vi "Burning Queue.vi"() -> (0 "error out 2":errorcluster)   [LabVIEW 2022 SP3]
uses:
  Type Def/Burning States.ctl
panel:
  in  "error in (no error)":errorcluster
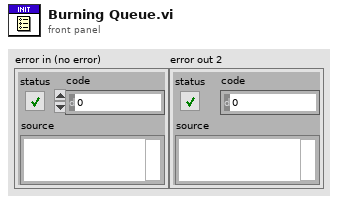
[diagram p1: front panel]
types:
  T1 = typedef "Burning States.ctl" = enum16{"Open Ports", "Close Ports", "Main", "Settings", "Voltaje", "Probe", "Lenguaje", "Callibration", "Exit", "Voltage Test", "Test 2", "End test"}
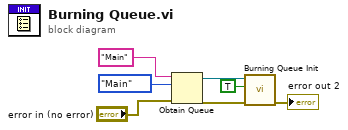
[diagram p0: block diagram]
diagram:
  n1 = Obtain Queue(name (unnamed)="Main", element data type=Burning_States."Main", error in (no error)="error in (no error)") -> (queue out=w4:refnum<queue>, error out=w3:errorcluster)  [unwired: 2 in, 1 out]
  n2 = call "Burning Queue Init.vi"("error in (no error) 2"=w3, "Read:F/Wirte:T"=TRUE, "queue out"=w4) -> ("error out 2"=→"error out 2":errorcluster)  [unwired: 7 in, 1 out]
